vi "Time Estimate.vi"(8 "error in (no error)":errorcluster, 9 "expmode":i32, 10 "scantype":T1(ring), 11 "Scanner.lvclass":refnum<class "Scanner.lvclass">) -> (0 "error out":errorcluster, 1 "Time Estimate":string, 2 "time":dbl[unit], 3 "Scanner.lvclass out":refnum<class "Scanner.lvclass">)   [LabVIEW 2009, in "Scanner.lvclass"]
doc: "(Dynamic) Return an estimate of the time remaining to scan over this Scanner's preconfigured Range."
uses:
  Scanner.lvclass
  Global/Set Up.vi
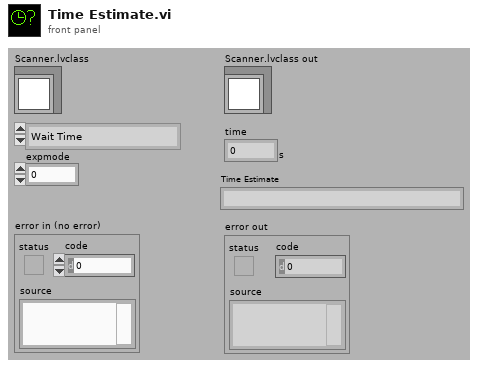
[diagram p1: front panel]
types:
  T1 = enum16{"Wait Time", "Pulse Width", "Wavelength", "Magnetic Field", "rf Scan"}
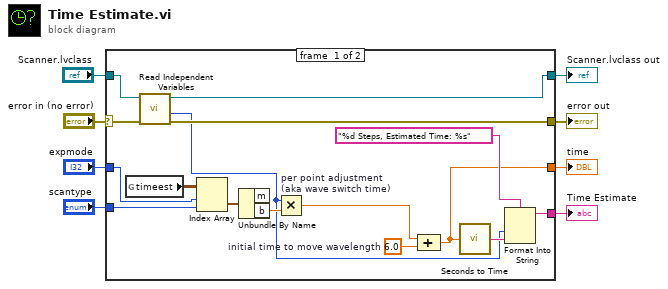
[diagram p0: block diagram]
diagram:
  n1 = case shown="No Error" "error in (no error)" {
    selector: "error in (no error)" -> [w16 w25]
    tunnel: [w11 _] -> w1
    tunnel: "expmode" -> [w23 _]
    tunnel: "scantype" -> [w17 _]
    tunnel: [w9 _] -> w6
    tunnel: [w18 w26] -> w4
    tunnel: "Scanner.lvclass" -> [w19 w26]
    tunnel: [w20 w25] -> w3
    frame #0 {
      w15 = dbl[unit] 6.0  # initial time to move wavelength
      n2 = global read "Set Up.vi" "timeest"() -> (w24:cluster{"m":dbl, "b":dbl[unit]}[][])
      n3 = call-dynamic "Read Independent Variables.vi"("error in (no error)"=w16, "Scanner.lvclass in"=w19) -> ("error out"=w20:errorcluster, "size"=w12:i32, "Scanner.lvclass out"=w18:refnum<class "Scanner.lvclass">)  [unwired: 7 out]
      n4 = Index Array(array=w24, index (row)=w23, index (col)=w17) -> (element=w22:cluster{"m":dbl, "b":dbl[unit]})
      n5 = Unbundle By Name(w22) -> ("b"=w21:dbl[unit])  [unwired: 1 out]
      n6 = Multiply "per point adjustment\n(aka wave switch time)"(x=w12, y=w21) -> (x*y=w10:dbl[unit])
      n7 = Compound Arithmetic op=ADD(w10, w15) -> (w9:dbl[unit])
      n8 = call "Seconds to Time.vi"("Seconds"=w9) -> ("Time"=w13:string)
      n9 = Format Into String(format string="%d Steps, Estimated Time: %s", w12, w13) -> (resulting string=w11:string)  [unwired: 2 in, 1 out]
    }
    frame #1 {
    }
  }
  "time" <- w6
  "Scanner.lvclass out" <- w4
  "error out" <- w3
  "Time Estimate" <- w1
